vi "Sequence-DefaultStyle.vi"(8 "error in (no error)":errorcluster, 10 "Test Steps":string[](array[string]), 11 "MCListbox Refnum":refnum<vi>) -> (0 "error out":errorcluster, 3 "MCListbox Refnum(dup)":refnum<vi>)   [LabVIEW 2020, in "CSMStand(Lite).lvlib"]
uses:
  CSMStand(Lite).lvlib
  <vilib>/Utility/miscctls.llb/LVRowAndColumnUnsignedTypeDef.ctl
  <vilib>/Utility/miscctls.llb/LVRowAndColumnTypeDef.ctl
  <userlib>/NEVSTOP-Programming-Palette/Dialog & Interface/_support/Autosize All MultiListbox Columns (Uniform Text)_nevstop.vi
  <vilib>/regexp/Match Regular Expression.xnode
panel:
  # "Connector Pane"
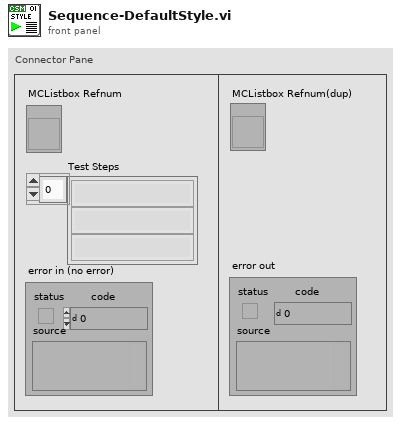
[diagram p1: front panel]
types:
  T1 = typedef "LVRowAndColumnTypeDef.ctl" = cluster{"Row":i32, "Column":i32}
  T2 = typedef "LVRowAndColumnUnsignedTypeDef.ctl" = cluster{"Row":u32, "Column":u32}
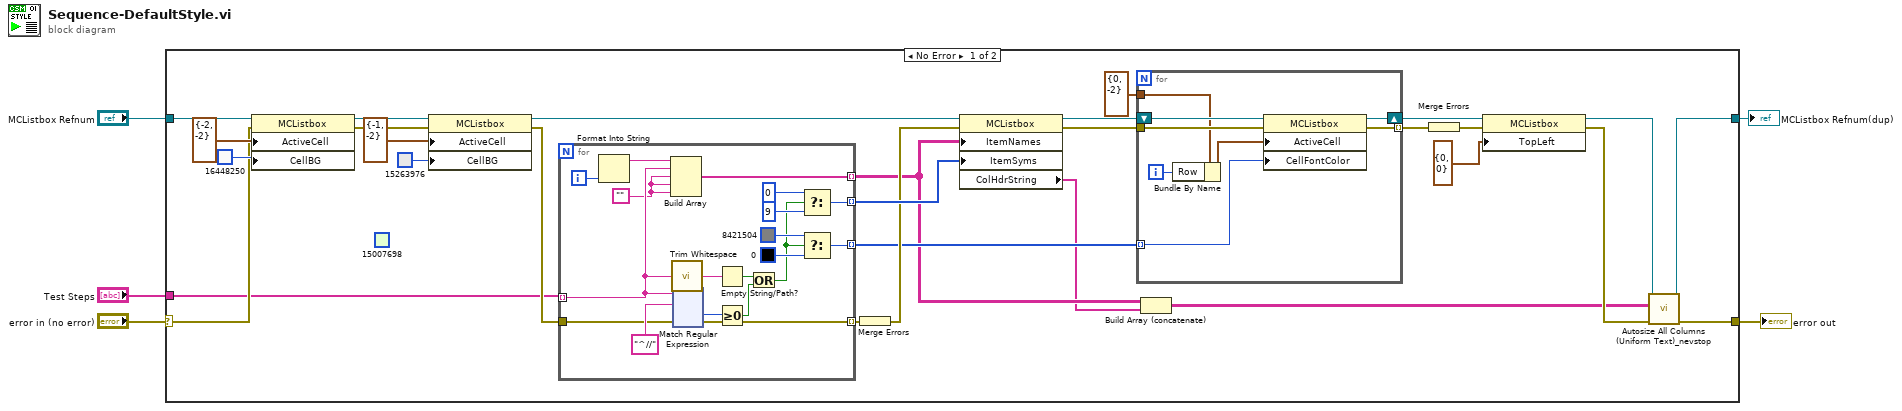
[diagram p0: block diagram]
diagram:
  n1 = case shown="No Error" "error in (no error)" {
    selector: "error in (no error)" -> [w11 w177]
    tunnel: [w29 w177] -> w5
    tunnel: "MCListbox Refnum" -> [w14 w176]
    tunnel: [w31 w176] -> w2
    tunnel: "Test Steps" -> [w10 _]
    frame No Error {
      (unwired) u32 15007698
      n2 = property class="MCListbox"(reference=w14, error in=w11, "ActiveCell"=T1 {"Row"=-2, "Column"=-2} ("Active Cell:Active Cell"), "CellBG"=u32 16448250) -> (reference out=w17:refnum<vi>, error out=w16:errorcluster)
      n3 = property class="MCListbox"(reference=w17, error in=w16, "ActiveCell"=T1 {"Row"=-1, "Column"=-2} ("Active Cell:Active Cell"), "CellBG"=u32 15263976) -> (reference out=w13:refnum<vi>, error out=w12:errorcluster)
      n4 = for {
        tunnel: w10 -> [w40] mode=indexing
        tunnel: [w51] -> w9 mode=indexing
        tunnel: [w43] -> w34 mode=indexing
        tunnel: w12 -> [w49]
        tunnel: [w48] -> w28 mode=indexing
        tunnel: [w44] -> w20 mode=indexing
        i -> [w53]
        w35 = ""
        n5 = Format Into String(w53) -> (resulting string=w52:string)  [unwired: 3 in, 1 out]
        n6 = Build Array(w52, w40, w35, w35, w35) -> (w51:string[])
        n7 = call <vilib>:"Trim Whitespace.vi"("string"=w40) -> ("trimmed string"=w39:string)  [unwired: 1 in]
        n8 = xnode "Match Regular Expression"("input string"=w40, "regular expression"="^//", "error in"=w49) -> ("offset past match"=w47:i32, "error out"=w48:errorcluster)  [unwired: 3 in, 3 out]
        n9 = Empty String/Path?(string/path=w39) -> (empty?=w38:bool)
        n10 = Greater Or Equal To 0?(x=w47) -> (x >= 0?=w37:bool)
        n11 = Or(x=w38, y=w37) -> (x .or. y?=w36:bool)
        n12 = Select(t=0, s=w36, f=9) -> (s? t:f=w43:i32)
        n13 = Select(t=u32 8421504 ("Active Cell:Cell Font:Color"), s=w36, f=u32 0 ("Active Cell:Cell Font:Color")) -> (s? t:f=w44:u32)
      }
      n14 = Merge Errors(w28) -> (w27:errorcluster)
      n15 = property class="MCListbox"(reference=w13, error in=w27, "ItemNames"=w9, "ItemSyms"=w34) -> (reference out=w26:refnum<vi>, error out=w25:errorcluster, "ColHdrString"=w8:string[])
      n16 = for {
        tunnel: w25 -> [w174]
        shift-right: [w173] -> w22
        shift-left: w26 -> [w175]
        tunnel: T1 {"Row"=0, "Column"=-2} ("Active Cell:Active Cell") -> [w170]
        tunnel: [w169] -> w23 mode=indexing
        tunnel: w20 -> [w168] mode=indexing
        i -> [w172]
        n17 = Bundle By Name(cluster=w170, "Row"=w172) -> (w171:T1)
        n18 = property class="MCListbox"(reference=w175, error in=w174, "ActiveCell"=w171, "CellFontColor"=w168) -> (reference out=w173:refnum<vi>, error out=w169:errorcluster)
      }
      n19 = Build Array (concatenate)(w9, w8) -> (w7:string[][])
      n20 = Merge Errors(w23) -> (w21:errorcluster)
      n21 = property class="MCListbox"(reference=w22, error in=w21, "TopLeft"=T2 {"Row"=0, "Column"=0} ("Top Left Visible Cell")) -> (reference out=w32:refnum<vi>, error out=w30:errorcluster)
      n22 = call-poly <userlib>:"Autosize All Columns (Uniform Text)_nevstop.vi"("error in (no error)"=w30, "Array"=w7, "Control in"=w32) -> ("error out"=w29:errorcluster, "Control in"=w31:refnum<vi>)  [unwired: 7 in]
    }
    frame Error {
    }
  }
  "error out" <- w5
  "MCListbox Refnum(dup)" <- w2
